vi "FPGANic.Read-Debug-FIFOs.vi"(8 "error in":errorcluster, 10 "Clear Debug FIFOs":bool, 11 "FPGA VI Reference In":refnum<k20>) -> (0 "error out":errorcluster, 3 "Debug Data":T1)   [LabVIEW 2018]
uses:
  <vilib>/Utility/error.llb/Error Cluster From Error Code.vi
  <vilib>/rvi/errors/niLvFpgaAdjustHostInterfaceError.vi
  <vilib>/Field R&D Services/Logger/Private/Manager.vi
  <vilib>/rvi/interface/nirviMethod/nirviMethod.xnode
  <vilib>/FPGAPlugInAG/Dynamic/niLvFpga_ReadFifo_Dynamic.vi
  <vilib>/rvi/errors/niLvFpgaMergeErrorWithErrorCode.vi
  <vilib>/Field R&D Services/Logger/Logger.lvlib
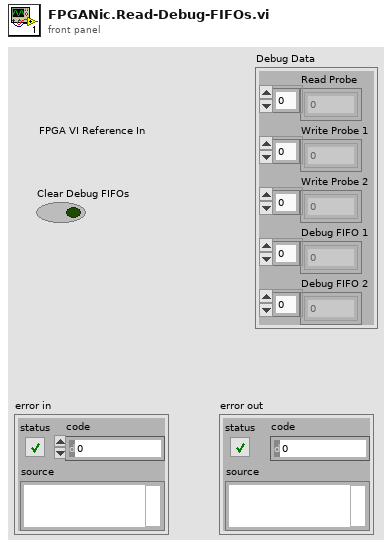
[diagram p1: front panel]
types:
  T1 = cluster{"Read Probe":u64[], "Write Probe 1":u64[], "Write Probe 2":u64[], "Debug FIFO 1":u32[], "Debug FIFO 2":u32[]}
  T2 = cluster{"Data":u64[], "Data":u64[], "Data":u64[], "Data":u32[], "Data":u32[]}
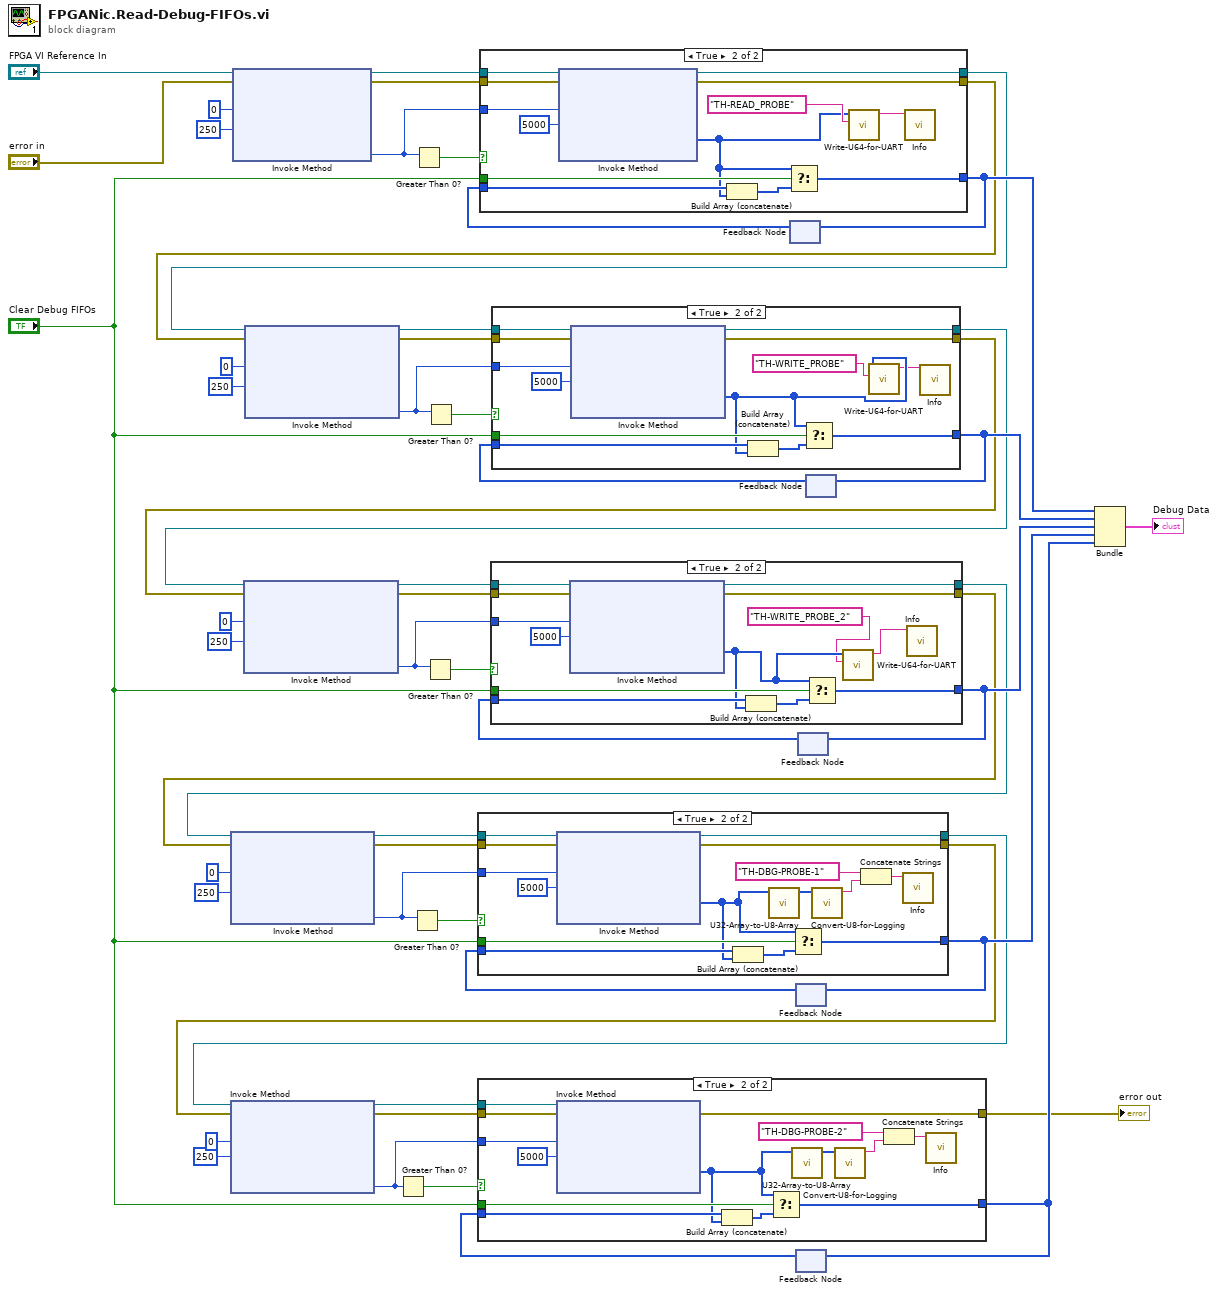
[diagram p0: block diagram]
diagram:
  n1 = xnode "Invoke Method"("FPGA VI Reference In"="FPGA VI Reference In", "error in"="error in", "Number of Elements"=u32 0, "Timeout (ms)"=250) -> ("FPGA VI Reference Out"=w38:refnum<k20>, "error out"=w37:errorcluster, "Elements Remaining"=w36:u32)  [unwired: 1 out]
  n2 = Greater Than 0?(x=w36) -> (x > 0?=w35:bool)
  n3 = feedback #1() -> (w39:u64[])  [unwired: 1 in]
  n4 = case shown="True" w35 {
    tunnel: w39 -> [w56 w69]
    tunnel: w36 -> [_ w68]
    tunnel: w37 -> [w55 w66]
    tunnel: w38 -> [w54 w65]
    tunnel: [w56 w62] -> w17
    tunnel: [w55 w64] -> w2
    tunnel: "Clear Debug FIFOs" -> [_ w61]
    tunnel: [w54 w60] -> w1
    frame False {
    }
    frame True {
      n5 = xnode "Invoke Method"("FPGA VI Reference In"=w65, "error in"=w66, "Number of Elements"=w68, "Timeout (ms)"=5000) -> ("FPGA VI Reference Out"=w60:refnum<k20>, "error out"=w64:errorcluster, "Data"=w58:u64[])  [unwired: 1 out]
      n6 = Build Array (concatenate)(w69, w58) -> (w63:u64[])
      n7 = Select(t=w58, s=w61, f=w63) -> (s? t:f=w62:u64[])
      n8 = call "Write-U64-for-UART.vi"("Log Message"="TH-READ_PROBE" ("string"), "Data"=w58) -> ("concatenated string"=w57:string)  [unwired: 9 in]
      n9 = call <vilib>:"Info.vi"("Message"=w57) -> ()  [unwired: 10 in, 1 out]
    }
  }
  n10 = xnode "Invoke Method"("FPGA VI Reference In"=w1, "error in"=w2, "Number of Elements"=u32 0, "Timeout (ms)"=250) -> ("FPGA VI Reference Out"=w45:refnum<k20>, "error out"=w44:errorcluster, "Elements Remaining"=w43:u32)  [unwired: 1 out]
  n11 = Greater Than 0?(x=w43) -> (x > 0?=w42:bool)
  n12 = feedback-in #1(w17) -> ()
  n13 = feedback #2() -> (w26:u32[])  [unwired: 1 in]
  n14 = feedback #3() -> (w20:u32[])  [unwired: 1 in]
  n15 = feedback #4() -> (w53:u64[])  [unwired: 1 in]
  n16 = feedback #5() -> (w46:u64[])  [unwired: 1 in]
  n17 = case shown="True" w42 {
    tunnel: w46 -> [w72 w85]
    tunnel: w43 -> [_ w84]
    tunnel: w44 -> [w71 w82]
    tunnel: w45 -> [w70 w81]
    tunnel: [w72 w78] -> w11
    tunnel: [w71 w80] -> w5
    tunnel: "Clear Debug FIFOs" -> [_ w77]
    tunnel: [w70 w76] -> w4
    frame False {
    }
    frame True {
      n18 = xnode "Invoke Method"("FPGA VI Reference In"=w81, "error in"=w82, "Number of Elements"=w84, "Timeout (ms)"=5000) -> ("FPGA VI Reference Out"=w76:refnum<k20>, "error out"=w80:errorcluster, "Data"=w74:u64[])  [unwired: 1 out]
      n19 = Build Array (concatenate)(w85, w74) -> (w79:u64[])
      n20 = Select(t=w74, s=w77, f=w79) -> (s? t:f=w78:u64[])
      n21 = call "Write-U64-for-UART.vi"("Log Message"="TH-WRITE_PROBE" ("string"), "Data"=w74) -> ("concatenated string"=w73:string)  [unwired: 9 in]
      n22 = call <vilib>:"Info.vi"("Message"=w73) -> ()  [unwired: 10 in, 1 out]
    }
  }
  n23 = xnode "Invoke Method"("FPGA VI Reference In"=w4, "error in"=w5, "Number of Elements"=u32 0, "Timeout (ms)"=250) -> ("FPGA VI Reference Out"=w52:refnum<k20>, "error out"=w51:errorcluster, "Elements Remaining"=w50:u32)  [unwired: 1 out]
  n24 = Greater Than 0?(x=w50) -> (x > 0?=w49:bool)
  n25 = case shown="True" w49 {
    tunnel: w53 -> [w88 w101]
    tunnel: w50 -> [_ w100]
    tunnel: w51 -> [w87 w98]
    tunnel: w52 -> [w86 w97]
    tunnel: [w88 w94] -> w18
    tunnel: [w87 w96] -> w7
    tunnel: "Clear Debug FIFOs" -> [_ w93]
    tunnel: [w86 w92] -> w6
    frame False {
    }
    frame True {
      n26 = xnode "Invoke Method"("FPGA VI Reference In"=w97, "error in"=w98, "Number of Elements"=w100, "Timeout (ms)"=5000) -> ("FPGA VI Reference Out"=w92:refnum<k20>, "error out"=w96:errorcluster, "Data"=w91:u64[])  [unwired: 1 out]
      n27 = Build Array (concatenate)(w101, w91) -> (w95:u64[])
      n28 = Select(t=w91, s=w93, f=w95) -> (s? t:f=w94:u64[])
      n29 = call "Write-U64-for-UART.vi"("Log Message"="TH-WRITE_PROBE_2" ("string"), "Data"=w91) -> ("concatenated string"=w89:string)  [unwired: 9 in]
      n30 = call <vilib>:"Info.vi"("Message"=w89) -> ()  [unwired: 10 in, 1 out]
    }
  }
  n31 = xnode "Invoke Method"("FPGA VI Reference In"=w6, "error in"=w7, "Number of Elements"=u32 0, "Timeout (ms)"=250) -> ("FPGA VI Reference Out"=w27:refnum<k20>, "error out"=w28:errorcluster, "Elements Remaining"=w29:u32)  [unwired: 1 out]
  n32 = Greater Than 0?(x=w29) -> (x > 0?=w30:bool)
  n33 = case shown="True" w30 {
    tunnel: w26 -> [w104 w119]
    tunnel: w29 -> [_ w118]
    tunnel: w28 -> [w103 w116]
    tunnel: w27 -> [w102 w115]
    tunnel: [w104 w112] -> w12
    tunnel: [w103 w114] -> w9
    tunnel: "Clear Debug FIFOs" -> [_ w111]
    tunnel: [w102 w110] -> w8
    frame False {
    }
    frame True {
      n34 = xnode "Invoke Method"("FPGA VI Reference In"=w115, "error in"=w116, "Number of Elements"=w118, "Timeout (ms)"=5000) -> ("FPGA VI Reference Out"=w110:refnum<k20>, "error out"=w114:errorcluster, "Data"=w105:u32[])  [unwired: 1 out]
      n35 = Build Array (concatenate)(w119, w105) -> (w113:u32[])
      n36 = call "U32-Array-to-U8-Array.vi"("U32 [] in"=w105) -> ("U8 [] out"=w109:u8[])  [unwired: 10 in]
      n37 = Select(t=w105, s=w111, f=w113) -> (s? t:f=w112:u32[])
      n38 = call "Convert-U8-for-Logging.vi"("u8 Array"=w109) -> ("Output String"=w108:string)  [unwired: 10 in]
      n39 = Concatenate Strings("TH-DBG-PROBE-1" ("string"), w108) -> (w107:string)
      n40 = call <vilib>:"Info.vi"("Message"=w107) -> ()  [unwired: 10 in, 1 out]
    }
  }
  n41 = xnode "Invoke Method"("FPGA VI Reference In"=w8, "error in"=w9, "Number of Elements"=u32 0, "Timeout (ms)"=250) -> ("FPGA VI Reference Out"=w23:refnum<k20>, "error out"=w22:errorcluster, "Elements Remaining"=w19:u32)  [unwired: 1 out]
  n42 = Greater Than 0?(x=w19) -> (x > 0?=w21:bool)
  n43 = case shown="True" w21 {
    tunnel: w20 -> [w121 w135]
    tunnel: w19 -> [_ w134]
    tunnel: w22 -> [w120 w132]
    tunnel: w23 -> [_ w131]
    tunnel: [w121 w128] -> w13
    tunnel: [w120 w130] -> w3
    tunnel: "Clear Debug FIFOs" -> [_ w127]
    frame False {
    }
    frame True {
      n44 = xnode "Invoke Method"("FPGA VI Reference In"=w131, "error in"=w132, "Number of Elements"=w134, "Timeout (ms)"=5000) -> ("error out"=w130:errorcluster, "Data"=w122:u32[])  [unwired: 2 out]
      n45 = Build Array (concatenate)(w135, w122) -> (w129:u32[])
      n46 = Select(t=w122, s=w127, f=w129) -> (s? t:f=w128:u32[])
      n47 = call "U32-Array-to-U8-Array.vi"("U32 [] in"=w122) -> ("U8 [] out"=w126:u8[])  [unwired: 10 in]
      n48 = call "Convert-U8-for-Logging.vi"("u8 Array"=w126) -> ("Output String"=w125:string)  [unwired: 10 in]
      n49 = Concatenate Strings("TH-DBG-PROBE-2" ("string"), w125) -> (w124:string)
      n50 = call <vilib>:"Info.vi"("Message"=w124) -> ()  [unwired: 10 in, 1 out]
    }
  }
  "error out" <- w3
  n51 = feedback-in #2(w12) -> ()
  n52 = feedback-in #3(w13) -> ()
  n53 = feedback-in #4(w18) -> ()
  n54 = feedback-in #5(w11) -> ()
  n55 = Bundle("Data"=w17, "Data"=w11, "Data"=w18, "Data"=w12, "Data"=w13) -> (→"Debug Data":T2)  [unwired: 1 in]
